vi "demo - long bad VI.vi"() -> ()   [LabVIEW 2024]
uses:
  <vilib>/Instr/_visa.llb/VISA Configure Serial Port (Instr).vi
  <vilib>/Utility/sysdir.llb/System Directory Type.ctl
  <vilib>/Analysis/NI_AALBase.lvlib
  <resource>/objmgr/daqmx.rc
  <vilib>/Utility/error.llb/DialogType.ctl
  <vilib>/sound2/lvsound2.llb/Sampling Mode.ctl
  <vilib>/sound2/lvsound2.llb/Sound Data Format.ctl
  <instrlib>/niScope/Configure/Trigger/niScope Configure Trigger Immediate.vi
  <instrlib>/niScope/Configure/Trigger/niScope Configure Trigger Digital.vi
  <instrlib>/niScope/Configure/Trigger/niScope Configure Trigger Edge.vi
  <instrlib>/niScope/Acquire/niScope Multi Read Cluster.vi
  <vilib>/Analysis/1siggen.llb/Ramp Pattern by Samples.vi
  <vilib>/DAQmx/create/channels.llb/DAQmx Create Channel (AI-Voltage-Basic).vi
  <vilib>/sound2/lvsound2.llb/Sound Output Set Volume (Single).vi
  <vilib>/DAQmx/read.llb/DAQmx Read (Analog 1D Wfm NChan NSamp).vi
  <vilib>/sound2/lvsound2.llb/Sound Output Write (DBL Single).vi
  <vilib>/DAQmx/configure/timing.llb/DAQmx Timing (Sample Clock).vi
  <vilib>/Utility/traverseref.llb/VI Scripting - Traverse.lvlib
  <vilib>/Utility/traverseref.llb/TRef TravTarget.ctl
  Serial - Settings.ctl
panel:
  out "Word count as text:":string
  out "Map of word to occurrence count:":map{string, u64}(c390)
  in  "Ignore these words:":string[](array[string])=["the", "an", "a"]
  in  "Count the words in this text:":string="Macbeth by William Shakespeare\nTomorrow, and tomorrow, and tomorrow,\nCreeps in this petty pace from day to day\nTo the last syllable of recorded time,\nAnd all our yesterdays have lighted fools\nThe way to dusty death. Out, out, brief candle!\nLife's but a walking shadow, a poor player\nThat struts and frets his hour upon the stage\nAnd then is heard no more: it is a tale\nTold by an idiot, full of sound and fury,\nSignifying nothing."
  in  "Tab Control 2":T1(tab)
  out "Numeric Result":bool
  in  "Numeric 2":i32=1
  in  "Numeric 1":i32=1
  out "String Result":bool
  in  "String 2":string="labview"
  in  "String 1":string="LabVIEW"
  out "Path Result":bool
  in  "Path 2":path=path "C:/TEST.TXT"
  in  "Path 1":path=path "c:/test.txt"
  out "Cluster Result":T2
  in  "Cluster 2":T3={"String"="test", "Numeric"=3.0, "Boolean"=TRUE}
  in  "Cluster 1":T3={"String"="test", "Numeric"=3.0, "Boolean"=TRUE}
  out "Numeric Refnum Value 2":u32
  out "Numeric Refnum Value 1":u32
  out "Refnum Result":bool
  in  "Time Stamp":timestamp
  out "Array to Scalar Result":bool[](array[boolean])
  in  "Scalar":dbl=2.0
  in  "Array":dbl[](array[numeric])=[1.0, 2.0, 3.0]
  out "Array to Array Result":bool[](array[boolean])
  in  "Array to Array 2":dbl[](array[numeric])=[1.0, 2.0, 3.0]
  in  "Array to Array 1":dbl[](array[numeric])=[1.0, 2.0, 3.0]
  in  "Tab Control":T4(tab)
  out "Max of X and Y":i32
  out "Min of X and Y":i32
  in  "Numeric Y":i32=56
  in  "Numeric X":i32=45
  out "Min String":string
  out "Max String":string
  in  "String Y":string="test ABC"
  in  "String X":string="test D"
  out "Min Path":path
  out "Max Path":path
  in  "Path Y":path=path "C:/Test1234"
  in  "Path X":path=path "C:/Test2"
  out "Maximum Cluster":T5
  out "Minimum Cluster":T5
  in  "Input Cluster Y":T5={"Numeric"=0.0, "String"="VI", "Numeric 2"=7.0}
  in  "Input Cluster X":T5={"Numeric"=1.0, "String"="test", "Numeric 2"=-3.0}
  out "Earliest Time":timestamp
  out "Latest Time":timestamp
  in  "Time Stamp Y":timestamp=timestamp(2327499010.485 s since 1904-01-01)
  in  "Time Stamp X":timestamp=timestamp(3084908797.174 s since 1904-01-01)
  out "Min Array":dbl[](array[numeric])
  out "Max Array":dbl[](array[numeric])
  in  "Array Y":dbl[](array[numeric])=[1.0, 2.0, 3.0, 4.0]
  in  "Array X":dbl[](array[numeric])=[5.0, 4.0, 3.0, 2.0, 1.0]
  in  "Device ID":u32
  in  "Stop 5":bool
  in  "Frequency":dbl=500.0
  out "Generated Sound":waveform(dbl)(graph)
  in  "Volume":dbl(slide)=50.0 scale=0.0..100.0
  in  "Server Closed":string="The server VI closed the connection."
  in  "Stop 4":bool
  out "Waveform Graph 5":dbl[](graph)
  in  "Number of Samples":i32=10000
  in  "Sample Rate":dbl=10000.0
  in  "Sample Clock Source":tag="OnboardClock"
  in  "Max Voltage":dbl=5.0
  in  "Min Voltage":dbl=-5.0
  in  "Physical Channel":tag="6363_sim/ai0"
  out "Actual Sample Rate 2":dbl=1000.0 format="%0.2f"
  out "Waveform Graph 4":waveform(dbl)[](graph)
  in  "Stop 3":bool
  out "Waveform Graph 3":dbl[](graph)
  out "current iteration 2":i32
  out "Waveform Graph 2":dbl[](graph)
  out "current iteration":i32
  out "Option String":string
  in  "Vertical Noise \n(% Range)":dbl=4.0 format="%.2f"
  in  "Board Type":u16(ring)=1 items=["PCI", "PXI", "PXIe", "USB", "AT", "PCMCIA"]
  in  "Model":u16(ring)=3 items=["NI-5102", "NI-5105", "NI-5112", "NI-5114", "NI-5122", "NI-5124", "NI-5132", "NI-5133", "NI-5142", "NI-5152", "NI-5153", "NI-5154", "NI-5160 (2CH)", "NI-5160 (4CH)", "NI-5162 (2CH)", "NI-5162 (4CH)", "NI-5170R (4CH)", "NI-5170R (8CH)", "NI-5171R (8CH)", "NI-5185", "NI-5186", "NI-5620", "NI-5621", "NI-5622", "NI-5911", "NI-5922"]
  in  "Simulate":bool
  in  "Channel(s)":string="0,1"
  in  "Vertical Range (V)":dbl=5.0 format="%.2f"
  in  "Min. Sample Rate":dbl=1000000.0 step=1000000.0 format="%#.3p"
  in  "Min. Record Length":i32=1000
  out "Waveform Graph":T6(graph)
  out "Actual Record Length":i32=1000
  out "Actual Sample Rate":dbl format="%#.3p"
  in  "Trigger Type":u16(ring)=2 items=["Edge", "Digital", "Immediate"]
  in  "Input Impedance":u32(ring) items=["1 mega ohm", "75 ohms", "50 ohms"]
  in  "Max. Input Frequency (Hz)":dbl caption="Max. Input\nFrequency (Hz)" format="%.2f"
  in  "Ref Position":dbl=50.0 format="%.1f"
  in  "Trigger Slope":i32(ring) items=["Positive", "Negative"]
  in  "Trigger Level (V)":dbl format="%.2f"
  in  "Number Of Records":i32=1 step=1
  in  "Stop 2":bool caption="stop"
  in  "Trigger Source":string(combo)="0"
  in  "Vertical Coupling":i32(ring) items=["AC", "DC", "Ground"]
  in  "Resource Name":refnum<k15>="Dev1" caption="Resource Name(s)"
  in  "Current Temperature":dbl
  in  "Threshold":dbl
  out "Alarm":bool
  out "Waveform Chart":dbl(graph)
  in  "Stop":bool
  out "XY Graph 2":cluster{"Ramp Pattern":dbl[], dbl[]}(graph)
  in  "All data":dbl[][](array[numeric])=[[-10.0, -204.0, 492.55], [-9.0, -132.17359, 359.580355], [-8.0, -87.56192, 252.88208], [-7.0, -58.99533, 169.671655], [-6.0, -39.66976, 107.11768], [-5.0, -25.71875, 62.346875], [-4.0, -15.13824, 32.45008], [-3.0, -7.01377, 14.488255], [-2.0, -0.99968, 5.49848], [-1.0, 3.00009, 2.499955], [0.0, 5.0, 2.5], [1.0, 5.00011, 2.500055], [2.0, 3.00288, -0.49832], [3.0, -0.97003, -9.487445], [4.0, -6.81056, -27.44752], [5.0, -14.15625, -57.340625], [6.0, -22.07104, -102.10472], [7.0, -28.52447, -164.647645], [8.0, -29.61888, -247.84112], [9.0, -18.51421, -354.514745]]
  out "Data written to":path
  out "XY Graph":cluster{"x axis":dbl[], "plot 1":dbl[]}[](graph)
  out "output cluster":T7
  out "timestamp":timestamp
  out "firmware":string
  out "array data":string[](array[string])
  in  "Serial Settings 2":T8={"baud rate"=9600, "data bits"=8, "parity"=enum."None", "stop bits"=10, "flow control"=0} {"flow control" items=["None"=0, "XON/XOFF"=1, "RTS/CTS"=2, "DTR/DSR"=4]; "stop bits" items=["1.0"=10, "1.5"=15, "2.0"=20]; "data bits" min=5 max=8 step=1; "baud rate" items=["75"=75, "110"=110, "134"=134, "150"=150, "300"=300, "600"=600, "1200"=1200, "1800"=1800, "2400"=2400, "4800"=4800, "7200"=7200, "9600"=9600, "14400"=14400, "19200"=19200, "28800"=28800, "38400"=38400, "56000"=56000, "57600"=57600, "115200"=115200, "128000"=128000, "230400"=230400]}
  out "bytes read 2":u32
  out "Response 2":string
  in  "delay before read (ms) 2":u32=500
  in  "VISA resource name 2":refnum<visa-resource-name>="COM3"
  in  "Serial Settings":T8={"baud rate"=9600, "data bits"=8, "parity"=enum."None", "stop bits"=10, "flow control"=0} {"flow control" items=["None"=0, "XON/XOFF"=1, "RTS/CTS"=2, "DTR/DSR"=4]; "stop bits" items=["1.0"=10, "1.5"=15, "2.0"=20]; "data bits" min=5 max=8 step=1; "baud rate" items=["75"=75, "110"=110, "134"=134, "150"=150, "300"=300, "600"=600, "1200"=1200, "1800"=1800, "2400"=2400, "4800"=4800, "7200"=7200, "9600"=9600, "14400"=14400, "19200"=19200, "28800"=28800, "38400"=38400, "56000"=56000, "57600"=57600, "115200"=115200, "128000"=128000, "230400"=230400]}
  out "bytes read":u32
  out "Response":string
  in  "delay before read (ms)":u32=500
  in  "VISA resource name":refnum<visa-resource-name>="COM3"
  # "Equal? will return TRUE if both numerics are the same value."
  # "Equal? will return TRUE if both strings are the same value. The comparison is case-sensitive, so 'LabVIEW' and 'labview' would not be considered equal."
  # "Equal? will return TRUE if both paths are the same value. The comparison is case-insensitive on some platforms (like Windows), and case-sensitive on other platforms (like Linux)."
  # "Equal? will return a cluster of Booleans with the same number of elements as the input clusters. Each Boolean will be TRUE if the corresponding elements in the clusters are the same value."
  # "Equal? will return TRUE if both refnums refer to the same control. This is the case, even if the refnums have different numeric values."
  # "Note: Control references from different sources are used for the refnum comparison. The actual value of this Time Stamp is not used in this example."
  # "When comparing arrays with arrays, Equal? will return an array of Booleans with the same number of elements as the smaller of the two input arrays. When comparing an array to a scalar, Equal? will return an array of Booleans with the same number of elements as the array."
  # "Max & Min finds the maximum and minimum of two numeric values."
  # "Max & Min compares the two strings character by character until it finds a character that has a higher ASCII numeric value. String length is not taken into account."
  # "Max & Min compares the two paths character by character until it finds a character that has a higher ASCII numeric value. Path length is not taken into account."
  # "Max & Min compares the clusters element by element, and returns clusters of the comparison results. The resulting clusters will have the same data type as the input clusters."
  # "Max & Min finds the latest time (maximum) and earliest time (minimum) of two time stamp values."
  # "Max & Min compares the arrays element by element, and returns arrays of the comparison results. The resulting arrays will be the same size as the smaller of the two input arrays."
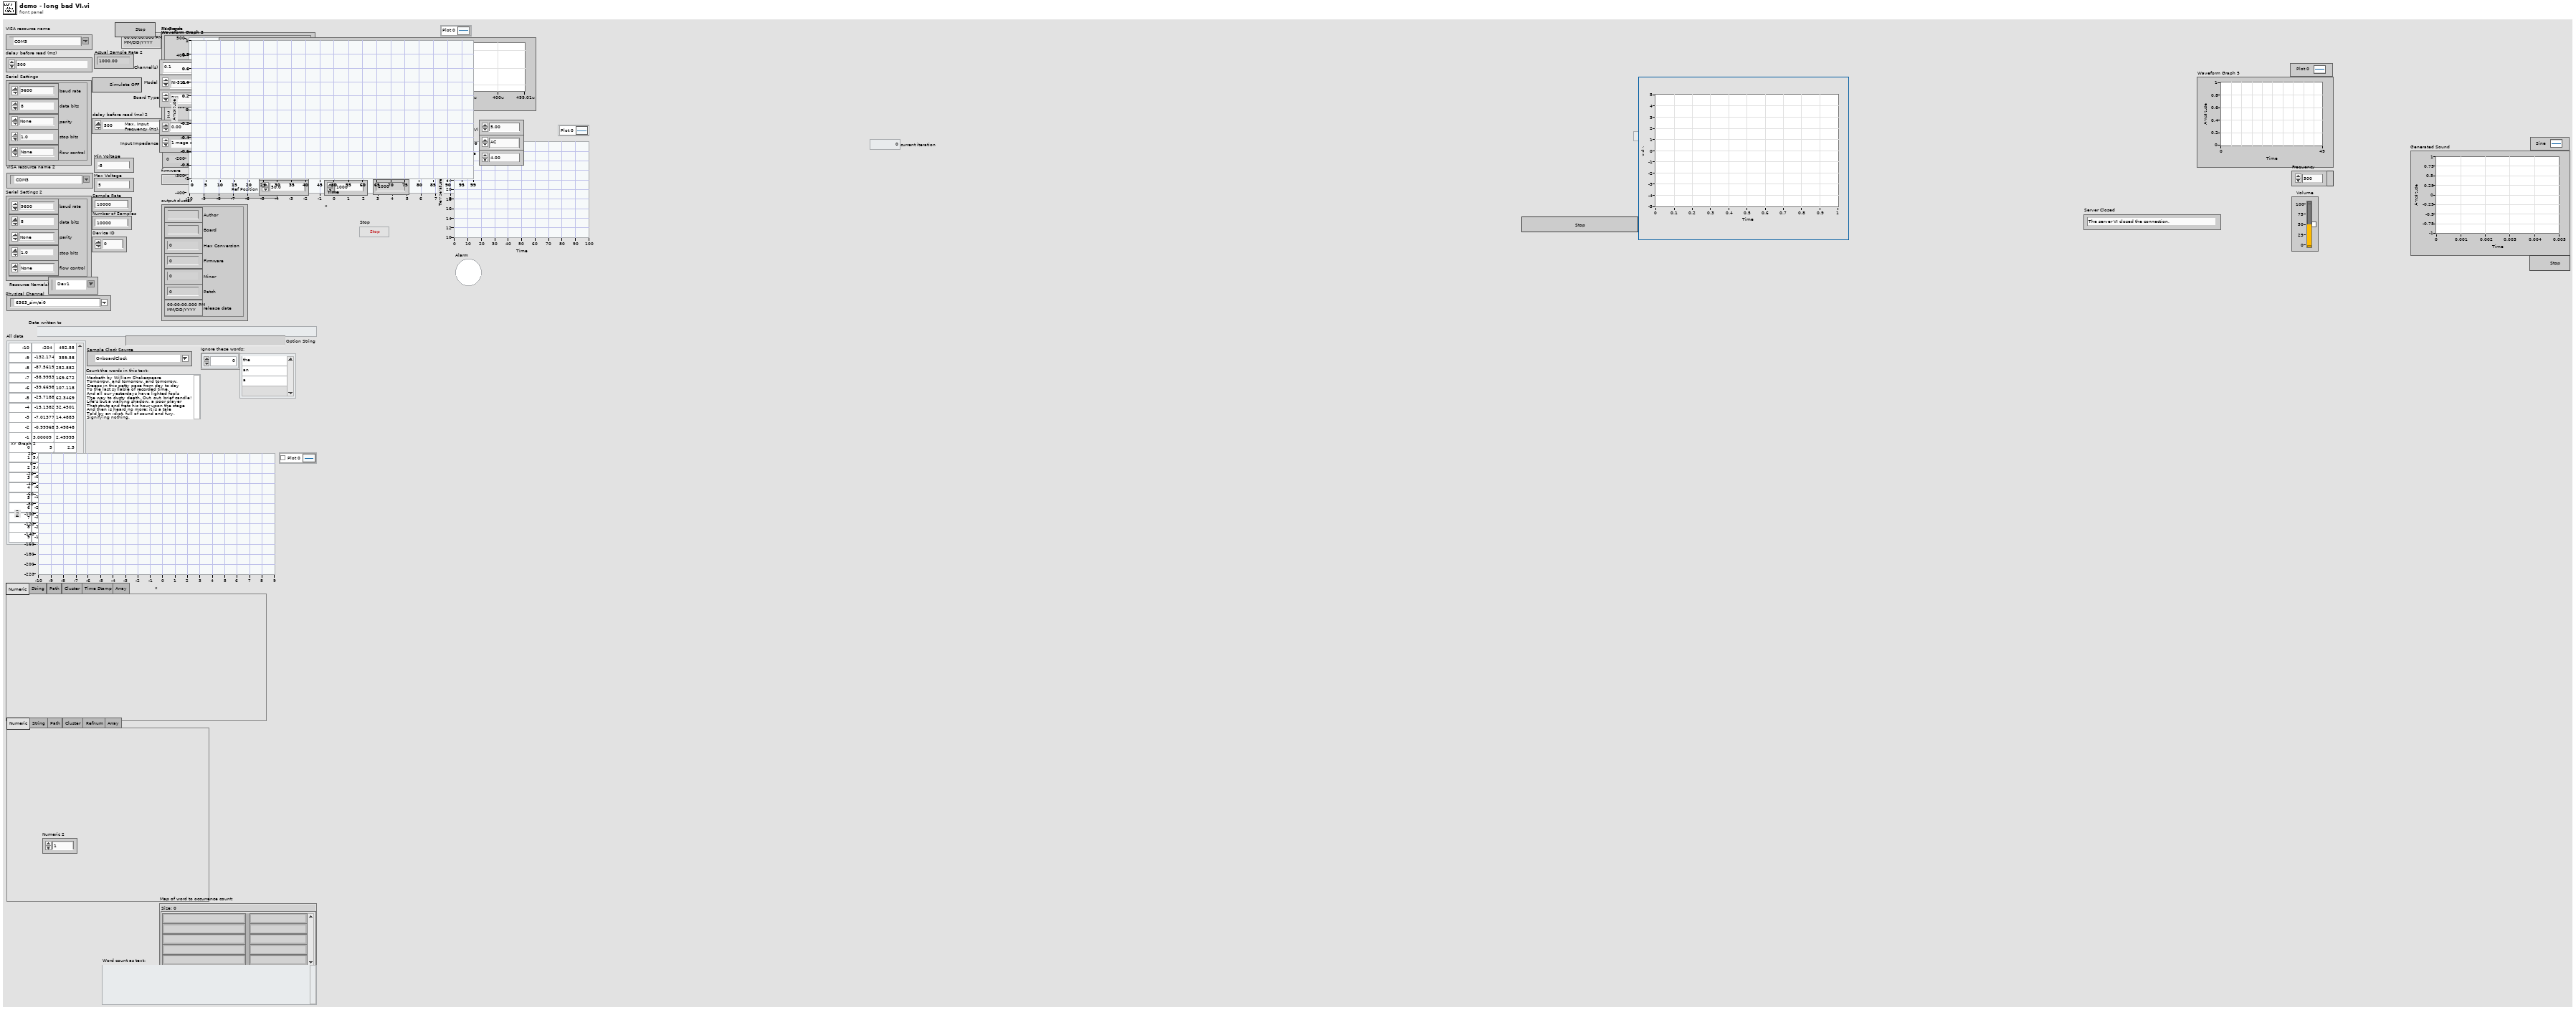
[diagram p1: front panel]
types:
  T1 = enum32{"Numeric", "String", "Path", "Cluster", "Refnum", "Array"}
  T2 = cluster{"String":bool, "Numeric":bool, "Boolean":bool}
  T3 = cluster{"String":string, "Numeric":dbl, "Boolean":bool}
  T4 = enum32{"Numeric", "String", "Path", "Cluster", "Time Stamp", "Array"}
  T5 = cluster{"Numeric":dbl, "String":string, "Numeric 2":dbl}
  T6 = cluster{"relativeInitialX":dbl, "xIncrement":dbl, "wfm":dbl[]}[]
  T7 = cluster{"Author":string, "Board":string, "Hex Conversion":u32, "Firmware":i32, "Minor":i32, "Patch":i32, "release date":timestamp}
  T8 = typedef "Serial - Settings.ctl" = cluster{"baud rate":u32, "data bits":u16, "parity":enum16{"None", "Odd", "Even", "Mark", "Space"}, "stop bits":u16, "flow control":u16}
  T9 = typedef "Sound Data Format.ctl" = cluster{"sample rate (S/s)":dbl, "number of channels":i32, "bits per sample":i32}
  T10 = typedef "TRef TravTarget.ctl" = enum16{"FP", "BD", "Other"}
  T11 = enum32{"Modify Entry only if found", "Add or Modify Entry", "Delete Entry"}
  T12 = enum16{"open", "replace", "create", "open or create", "replace or create", "replace or create with confirmation"}
  T13 = typedef "System Directory Type.ctl" = i32
  T14 = cluster{string, string, u32, i32, i32, i32, timestamp}
  T15 = typedef "DialogType.ctl" = u16
  T16 = typedef "Sampling Mode.ctl" = i32
  T17 = typedef "Sound Output Task ID.ctl" = u32
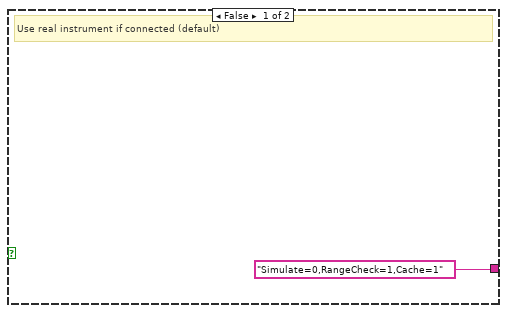
[diagram p2: hidden frame]
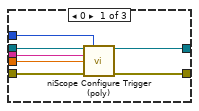
[diagram p3: hidden frame]
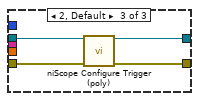
[diagram p4: hidden frame]
diagram:
  n1 = flat-sequence {
    frame #0 {
      w11 = "*IDN?\n"  # Command
      # "Report any Errors"
      # "Release Instrument"
      # "Read reply data on serial port"
      # "Wait for travel down cable"
      # "Send Command"
      # "Reserve and Configure Hardware"
      # "#vi_description \nSends a simple serial request and receives a response as as string of byte characters.\nModified NI Example.\nThetic Engineering Ltd."
      # "Use the VISA Configure Serial Port VI to configure the serial port. Send the \"*IDN?\" command with the VISA Write function. Read the response from the instrument with the VISA Read function. Note that the \"Bytes at Port\" property is used to determine how much data to read. For a single read use case, this is acceptable. For a continuous serial read, a more general approach is recommended. For an example of how to perform continuous serial communication in a loop, open the Continuous Serial Write and Read.vi in the same folder as this example."
      n2 = Unbundle By Name("Serial Settings") -> ("baud rate"=w5:u32, "data bits"=w4:u16, "parity"=w3:enum16{"None", "Odd", "Even", "Mark", "Space"}, "stop bits"=w2:u16, "flow control"=w1:u16)
      n3 = call-poly "VISA Configure Serial Port"("VISA resource name"="VISA resource name", "baud rate (9600)"=w5, "data bits (8)"=w4, "parity (0:none)"=w3, "stop bits (10: 1 bit)"=w2, "flow control (0:none)"=w1) -> ("VISA resource name out"=w20:refnum<visa-resource-name>, "error out"=w21:errorcluster)  [unwired: 3 in, 5 out]
      n4 = VISA Write(VISA resource name=w20, write buffer=w11, error in (no error)=w21) -> (VISA resource name out=w14:refnum<visa-resource-name>, error out=w16:errorcluster)  [unwired: 1 out]
      n5 = flat-sequence {
        tunnel: w16 -> [w24]
        tunnel: [w24] -> w15
        tunnel: w14 -> [w23]
        tunnel: [w23] -> w13
        tunnel: "delay before read (ms)" -> [w25]
        frame #0 {
          n6 = Wait (ms)(milliseconds to wait=w25) -> ()  [unwired: 1 out]
        }
      }
      n7 = property on="Property Node" class="Instr"(reference=w13, error in=w15) -> (reference out=w10:refnum<visa-resource-name>, error out=w9:errorcluster, "Serial Settings:Number of Bytes at Serial Port"=w7:u32)
      "bytes read" <- w7
      n8 = VISA Read(VISA resource name=w10, byte count=w7, error in (no error)=w9) -> (VISA resource name out=w18:refnum<visa-resource-name>, read buffer=→"Response":string, error out=w19:errorcluster)  [unwired: 1 out]
      n9 = VISA Close(VISA resource name=w18, error in (no error)=w19) -> (error out=w17:errorcluster)
      n10 = call <vilib>:"Simple Error Handler.vi"("error in (no error)"=w17) -> ()  [unwired: 1 in, 8 out]
    }
    frame #1 {
      w30 = 2  # column
      w31 = 1  # column
      w32 = 0  # column
      w34 = "x,function1,function2\n"  # header
      w36 = "data.csv"  # filename
      w37 = enum16{"read/write", "read-only", "write-only"}."write-only"  # access (0:read/write)
      w38 = T12."replace or create"  # operation (0:open)
      w40 = T13 1 items=["User Home"=0, "User Desktop"=1, "User Documents"=2, "User Application Data"=3, "User Preferences"=4, "User Temporary"=5, "Public Documents"=6, "Public Application Data"=7, "Public Preferences"=8, "Public Cache"=13, "System Core Libraries"=9, "System Installed Libraries"=10, "Application Files"=11, "Boot Volume Root"=12]  # system directory type
      w48 = ","  # delimiter
      w49 = "%.6f"  # format string
      # "Close the file"
      # "Write measurement data to the file, which is already a comma-separated table"
      # "Write the names of columns, at the first line, and then move the cursor to the next line"
      # "Create a file on the desktop with the right permissions and open it"
      # "Provide a 2D array (table) and convert all values to strings, separated by commas"
      # "Source data to plot of f(x) and x"
      # "#vi_description \nPlots a polynomial equation to an XY graph and stores the values into a text file.\nThetic Engineering Ltd."
      # "Create xy pairs and plot to XY graph"
      n11 = Index Array(array="All data", index (col) #1=w32, index (col) #2=w31, index (col) #3=w30) -> (element #1=w29:dbl[], element #2=w28:dbl[], element #3=w27:dbl[])  [unwired: 3 in]
      n12 = call <vilib>:"Get System Directory.vi"("system directory type"=w40) -> ("system directory"=w39:path)  [unwired: 10 in]
      n13 = Build Path(base path=w39, name or relative path=w36) -> (appended path=w33:path)
      "Data written to" <- w33
      n14 = Array To Spreadsheet String(delimiter (Tab)=w48, array="All data", 3:w49) -> (spreadsheet string=w47:string)
      n15 = Open/Create/Replace File(file path (use dialog)=w33, operation (0:open)=w38, access (0:read/write)=w37) -> (refnum out=w43:refnum<file>, error out=w44:errorcluster)  [unwired: 3 in, 1 out]
      n16 = Write to Text File(file (use dialog)=w43, text=w34, error in=w44) -> (refnum out=w45:refnum<file>, error out=w46:errorcluster)  [unwired: 1 in, 1 out]
      n17 = Write to Text File(file (use dialog)=w45, text=w47, error in=w46) -> (refnum out=w41:refnum<file>, error out=w42:errorcluster)  [unwired: 1 in, 1 out]
      n18 = Bundle("All data"=w29, "All data"=w28) -> (w52:cluster{"All data":dbl[], "All data":dbl[]})  [unwired: 1 in]
      n19 = Bundle("All data"=w29, "All data"=w27) -> (w51:cluster{"All data":dbl[], "All data":dbl[]})  [unwired: 1 in]
      n20 = Build Array(w52, w51) -> (→"XY Graph":cluster{"All data":dbl[], "All data":dbl[]}[])
      n21 = Close File(refnum=w41, error in=w42) -> (error out=w35:errorcluster)  [unwired: 1 out]
      n22 = call <vilib>:"Simple Error Handler.vi"("error in (no error)"=w35) -> ()  [unwired: 4 in, 5 out]
    }
    frame #2 {
      w53 = TRUE  # exclude end?
      w57 = 20  # samples
      w58 = 10.0  # end
      w59 = -10.0  # start
      # "#vi_description \nPlots a polynomial equation to an XY graph, demonstrating the use of a formula node.\nThetic Engineering Ltd."
      # "Create xy pairs and plot to XY graph"
      # "Generate integer values from -10 to 10"
      # "target equation (screenshot)"
      n23 = call-poly <vilib>:"Ramp Pattern.vi"("exclude end?"=w53, "start"=w59, "end"=w58, "samples"=w57) -> ("Ramp Pattern"=w55:dbl[])  [unwired: 6 in, 1 out]
      n24 = for {
        tunnel: w55 -> [w61] mode=indexing
        tunnel: [w60] -> w56 mode=indexing
        # "Auto-indexing For Loop will produce a result for each value of x"
        n25 = formula code="fx = 10**-5*x**7 + 10**-4*x**4 - x**2 + x + 5;"("x"=w61) -> ("fx"=w60:dbl)
      }
      n26 = Bundle("Ramp Pattern"=w55, w56) -> (→"XY Graph 2":cluster{"Ramp Pattern":dbl[], dbl[]})  [unwired: 1 in]
    }
    frame #3 {
      # "#vi_description \nChecks if temperature exceeds the threshold, in Celsius\nThetic Engineering Ltd."
      n27 = while {
        stop <- "Stop" stop-if-true
        w62 = u32 100  # millisecond multiple
        # "Checks if Temperature exceeds threshold, in Celsius"
        n28 = Wait Until Next ms Multiple(millisecond multiple=w62) -> ()  [unwired: 1 out]
        n29 = Greater Or Equal?(x="Current Temperature", y="Threshold") -> (x >= y?=→"Alarm":bool)
        "Waveform Chart" <- "Current Temperature"
      }
    }
    frame #4 {
      w74 = FALSE  # Reset Device
      # "#vi_description \nSimulates a 2 ch digitizer and plots the graph.  This is an NI example from NI-SCOPE that has been modifed.\nThetic Engineering Ltd."
      # "11"
      # "1. Form a string that will be used to initialize the oscilloscope. The simulation string should look like \"Simulate=1,DriverSetup=Model:5122;BoardType:PXI\".\n2. Open a session to the oscilloscope. Use init with options and pass the string formed in step 1.\n3. Configure the vertical parameters such as input range, offset and coupling.\n       For more information regarding channel names, refer to Channel String Syntax in the NI High-Speed Digitizers Help.\n4. Configure the channel characteristics such as input impedance and bandwidth.\n5. Configure the horizontal parameters such as sampling rate and number of samples to acquire.\n6. Configure the trigger. All oscilloscopes support immediate triggering. Choose between immediate, analog or digital.\n7. Use the Read function to Initiate the acquisition, wait until it finishes and fetch the acquired data. In simulation mode a Sine will be returned for channel 0 and a Square for channel 1.\n8. Query for the actual (coerced) record length.\n9. Query for the actual (coerced) sampling rate.\n10. Check for errors, and stop if any occurred. Also stop if the \"Stop\" button is clicked.\n11. Close the session and display any errors that might have occurred."
      # "2"
      n30 = case shown="True" "Simulate" {
        tunnel: ["Simulate=0,RangeCheck=1,Cache=1" ("option string") w91] -> w67
        frame False {
          # "Use real instrument if connected (default)"
        }
        frame True {
          (unwired) "BoardType:PCI"  # Board Type Format
          (unwired) "Model:5102;"  # Model String Format
          w94 = "Simulate=1,DriverSetup=Noise:"  # General Setup
          # "1"
          # "Generate option string to enable NI-SCOPE simulation"
          n31 = property on="Model" class="Ring (strict)"() -> ("Strings []"=w90:string[])  [unwired: 2 in, 2 out]
          n32 = property on="Board Type" class="Ring (strict)"() -> ("Strings []"=w82:string[])  [unwired: 2 in, 2 out]
          n33 = Index Array(array=w90, index="Model") -> (element=w88:string)
          n34 = Index Array(array=w82, index="Board Type") -> (element=w80:string)
          n35 = String Subset(string=w88, offset (0)=3 ("Offset (0)")) -> (substring=w85:string)  [unwired: 1 out]
          n36 = Concatenate Strings("BoardType:" ("Board Type Format"), w80) -> (w78:string)
          n37 = Concatenate Strings("Model:" ("String"), w85, ";" ("String")) -> (w86:string)
          n38 = Number To Fractional String(use system decimal point (T)=FALSE ("Use System Decimal Point (T)"), number="Vertical Noise \n(% Range)") -> (F-format string=w93:string)  [unwired: 2 out]
          n39 = Concatenate Strings(w94, w93, ";", w86, w78) -> (w91:string)
        }
      }
      "Option String" <- w67
      n40 = call <instrlib>:"niScope Initialize With Options.vi"("resource name"="Resource Name", "option string"=w67, "reset device"=w74) -> ("instrument handle"=w72:refnum<k15>, "error out"=w71:errorcluster)  [unwired: 2 in, 9 out]
      n41 = while {
        tunnel: w72 -> [w98]
        tunnel: [w104] -> w70
        shift-right: [w103] -> w69
        shift-left: w71 -> [w97]
        stop <- w105 stop-if-true
        # "10"
        # "9"
        # "8"
        # "6"
        # "7"
        # "5"
        # "4"
        # "3"
        n42 = call <instrlib>:"niScope Configure Vertical.vi"("instrument handle"=w98, "vertical coupling"="Vertical Coupling", "channels"="Channel(s)", "vertical range"="Vertical Range (V)", "error in"=w97) -> ("instrument handle out"=w123:refnum<k15>, "error out"=w122:errorcluster)  [unwired: 3 in, 6 out]
        n43 = call <instrlib>:"niScope Configure Chan Characteristics.vi"("instrument handle"=w123, "channels"="Channel(s)", "input impedance"="Input Impedance", "maximum input frequency"="Max. Input Frequency (Hz)", "error in"=w122) -> ("instrument handle out"=w120:refnum<k15>, "error out"=w121:errorcluster)  [unwired: 9 out]
        n44 = call <instrlib>:"niScope Configure Horizontal Timing.vi"("instrument handle"=w120, "number of records"="Number Of Records", "min sample rate"="Min. Sample Rate", "reference position"="Ref Position", "error in"=w121, "min record length"="Min. Record Length") -> ("instrument handle out"=w116:refnum<k15>, "error out"=w117:errorcluster)  [unwired: 1 in, 7 out]
        n45 = case "Trigger Selection" shown="1" "Trigger Type" {
          tunnel: w117 -> [w137 w143 w147]
          tunnel: [w133 w139 w144] -> w109
          tunnel: w116 -> [w136 w142 w146]
          tunnel: [w134 w140 w145] -> w110
          tunnel: "Trigger Source" -> [w135 w141 _]
          tunnel: "Trigger Level (V)" -> [w132 _ _]
          tunnel: "Trigger Slope" -> [w131 w138 _]
          frame 0 {
            n46 = call-poly <instrlib>:"niScope Configure Trigger (poly).vi"("instrument handle"=w136, "trigger slope"=w131, "trigger source"=w135, "trigger level"=w132, "error in"=w137) -> ("instrument handle out"=w134:refnum<k15>, "error out"=w133:errorcluster)  [unwired: 3 in, 6 out]
          }
          frame 1 {
            n47 = call-poly <instrlib>:"niScope Configure Trigger (poly).vi"("instrument handle"=w142, "trigger slope"=w138, "trigger source"=w141, "error in"=w143) -> ("instrument handle out"=w140:refnum<k15>, "error out"=w139:errorcluster)  [unwired: 2 in, 8 out]
          }
          frame 2, Default {
            n48 = call-poly <instrlib>:"niScope Configure Trigger (poly).vi"("instrument handle"=w146, "error in"=w147) -> ("instrument handle out"=w145:refnum<k15>, "error out"=w144:errorcluster)  [unwired: 12 out]
          }
        }
        n49 = call-poly <instrlib>:"niScope Read (poly).vi"("error in"=w109, "channels"="Channel(s)", "instrument handle"=w110) -> ("error out"=w107:errorcluster, "waveform"=→"Waveform Graph":T6, "instrument handle out"=w108:refnum<k15>)  [unwired: 2 in, 4 out]
        n50 = call <instrlib>:"niScope Actual Record Length.vi"("instrument handle"=w108, "error in"=w107) -> ("instrument handle out"=w127:refnum<k15>, "actual record length"=→"Actual Record Length":i32, "error out"=w126:errorcluster)  [unwired: 11 out]
        n51 = Wait (ms)(milliseconds to wait=u32 20 ("Milliseconds To Wait")) -> ()  [unwired: 1 out]
        n52 = call <instrlib>:"niScope Sample Rate.vi"("instrument handle"=w127, "error in"=w126) -> ("instrument handle out"=w104:refnum<k15>, "actual sample rate"=→"Actual Sample Rate":dbl, "error out"=w103:errorcluster)  [unwired: 11 out]
        n53 = Or(x=w103, y="Stop 2") -> (x .or. y?=w105:bool)
      }
      n54 = call <instrlib>:"niScope Close.vi"("instrument handle"=w70, "error in"=w69) -> ("error out"=w73:errorcluster)  [unwired: 13 out]
      n55 = call <vilib>:"Simple Error Handler.vi"("error in (no error)"=w73) -> ()  [unwired: 1 in, 8 out]
    }
    frame #5 {
      # "#vi_description \nPlot a finite sine wave onto a waveform graph\nThetic Engineering Ltd."
      n56 = for {
        N: 100 -> [_]
        tunnel: [w150] -> w148 mode=indexing
        i -> [w151]
        w152 = u32 10  # ms multiple
        w153 = 3  # y
        # "For Loop"
        n57 = Divide(x=w151, y=w153) -> (x/y=w154:dbl)
        n58 = Sine(x=w154) -> (sin(x)=w150:dbl)
        n59 = Wait Until Next ms Multiple(millisecond multiple=w152) -> ()  [unwired: 1 out]
        "current iteration" <- w151
      }
      "Waveform Graph 2" <- w148
    }
    frame #6 {
    }
    frame #7 {
      w164 = "%3s,%11s,%x,%1d.%1d.%1d.%<%Y%m%dT%H%M%S>T"  # format string
      w167 = "%<%Y%m%dT%H%M%S>T"  # format string
      w170 = "[0-9].[0-9].[0-9]."  # regular expression
      w172 = 3  # index
      w168 = ","  # delimiter
      w183 = "*IDN?\n"  # Command
      # "Single stage method"
      # "Multi-stage method"
      # "Report any Errors"
      # "Release Instrument"
      # "Read reply data on serial port"
      # "Wait for travel down cable"
      # "Send Command"
      # "Reserve and Configure Hardware"
      # "#vi_description \nSends a simple serial request and receives a response as as string of byte characters.\nModified NI Example.\nThetic Engineering Ltd."
      n60 = Unbundle By Name("Serial Settings 2") -> ("baud rate"=w178:u32, "data bits"=w177:u16, "parity"=w176:enum16{"None", "Odd", "Even", "Mark", "Space"}, "stop bits"=w175:u16, "flow control"=w174:u16)
      n61 = call-poly "VISA Configure Serial Port"("VISA resource name"="VISA resource name 2", "baud rate (9600)"=w178, "data bits (8)"=w177, "parity (0:none)"=w176, "stop bits (10: 1 bit)"=w175, "flow control (0:none)"=w174) -> ("VISA resource name out"=w192:refnum<visa-resource-name>, "error out"=w193:errorcluster)  [unwired: 3 in, 5 out]
      n62 = VISA Write(VISA resource name=w192, write buffer=w183, error in (no error)=w193) -> (VISA resource name out=w186:refnum<visa-resource-name>, error out=w188:errorcluster)  [unwired: 1 out]
      n63 = flat-sequence {
        tunnel: w188 -> [w196]
        tunnel: [w196] -> w187
        tunnel: w186 -> [w195]
        tunnel: [w195] -> w185
        tunnel: "delay before read (ms) 2" -> [w197]
        frame #0 {
          n64 = Wait (ms)(milliseconds to wait=w197) -> ()  [unwired: 1 out]
        }
      }
      n65 = property on="Property Node" class="Instr"(reference=w185, error in=w187) -> (reference out=w182:refnum<visa-resource-name>, error out=w181:errorcluster, "Serial Settings:Number of Bytes at Serial Port"=w180:u32)
      "bytes read 2" <- w180
      n66 = VISA Read(VISA resource name=w182, byte count=w180, error in (no error)=w181) -> (VISA resource name out=w190:refnum<visa-resource-name>, read buffer=w156:string, error out=w191:errorcluster)  [unwired: 1 out]
      "Response 2" <- w156
      n67 = call <vilib>:"Delimited String to 1D String Array.vi"("delimiter"=w168, "delimited string"=w156) -> ("string array"=w173:string[])  [unwired: 9 in]
      "array data" <- w173
      n68 = VISA Close(VISA resource name=w190, error in (no error)=w191) -> (error out=w189:errorcluster)
      n69 = Index Array "Index Array"(array=w173, index=w172) -> (element=w171:string)
      n70 = Match Pattern(string=w171, regular expression=w170) -> (match substring=→"firmware":string, after substring=w166:string)  [unwired: 1 in, 2 out]
      n71 = call <vilib>:"Simple Error Handler.vi"("error in (no error)"=w189) -> ()  [unwired: 1 in, 8 out]
      n72 = Scan From String "Scan From String"(format string=w167, input string=w166) -> (output 1=→"timestamp":timestamp)  [unwired: 3 in, 3 out]
      n73 = Scan From String "Scan From String"(format string=w164, input string=w156) -> (output 1=w163:string, output 2=w162:string, output 3=w161:u32, output 4=w160:i32, output 5=w159:i32, output 6=w158:i32, output 7=w157:timestamp)  [unwired: 9 in, 3 out]
      n74 = Bundle(w163, w162, w161, w160, w159, w158, w157) -> (→"output cluster":T14)  [unwired: 1 in]
    }
    frame #8 {
      # "#vi_description \nPlot a finite sine wave onto a waveform graph\nThetic Engineering Ltd."
      n75 = for {
        N: 100 -> [_]
        tunnel: [w200] -> w198 mode=indexing
        i -> [w201]
        w202 = u32 10  # ms multiple
        w203 = 3  # y
        # "For Loop"
        n76 = Divide(x=w201, y=w203) -> (x/y=w204:dbl)
        n77 = Sine(x=w204) -> (sin(x)=w200:dbl)
        n78 = Wait Until Next ms Multiple(millisecond multiple=w202) -> ()  [unwired: 1 out]
        "current iteration 2" <- w201
      }
      "Waveform Graph 3" <- w198
    }
    frame #9 {
      w215 = -1 items=["default"=-1, "RSE"=10083, "NRSE"=10078, "Differential"=10106, "Pseudodifferential"=12529]  # Terminal Configuration
      w205 = T15 3 items=["no dialog", "OK message", "continue or stop message", "OK message + warnings", "continue/stop + warnings"] ("type of dialog (OK msg:1)")
      w225 = 10123 items=["Finite Samples"=10178, "Continuous Samples"=10123, "Hardware Timed Single Point"=12522]  # Sample Mode
      # "#vi_description \nPlot buffered DAQmx data onto a waveform graph until the user presses stop or an error has occurred.\nThetic Engineering Ltd."
      # "Acquire Data"
      # "Timing Settings"
      # "Channel Settings"
      n79 = call-poly <vilib>:"DAQmx Create Virtual Channel.vi"("maximum value"="Max Voltage", "minimum value"="Min Voltage", "input terminal configuration"=w215, "physical channels"="Physical Channel") -> ("task out"=w223:refnum<k21>, "error out"=w224:errorcluster)  [unwired: 10 in]
      n80 = call-poly <vilib>:"DAQmx Timing.vi"("task/channels in"=w223, "sample mode"=w225, "samples per channel"="Number of Samples", "rate"="Sample Rate", "source"="Sample Clock Source", "error in"=w224) -> ("task out"=w227:refnum<k21>, "error out"=w226:errorcluster)  [unwired: 8 in]
      n81 = property class="DAQmx Timing"(reference=w227, error in=w226) -> (reference out=w222:refnum<k21>, error out=w221:errorcluster, "SampClk.Rate"=→"Actual Sample Rate 2":dbl)
      n82 = call <vilib>:"DAQmx Start Task.vi"("task/channels in"=w222, "error in"=w221) -> ("task out"=w220:refnum<k21>, "error out"=w219:errorcluster)  [unwired: 12 in]
      n83 = while {
        tunnel: w220 -> [w236]
        tunnel: w219 -> [w235]
        tunnel: [w234] -> w209
        tunnel: [w231] -> w208
        tunnel: "Number of Samples" -> [w228]
        stop <- w229 stop-if-true
        n84 = call-poly <vilib>:"DAQmx Read.vi"("task/channels in"=w236, "number of samples per channel"=w228, "error in"=w235) -> ("task out"=w234:refnum<k21>, "data"=→"Waveform Graph 4":waveform(dbl)[], "error out"=w231:errorcluster)  [unwired: 10 in]
        n85 = Unbundle By Name(w231) -> ("status"=w230:bool)
        n86 = Or(x=w230, y="Stop 3") -> (x .or. y?=w229:bool)
      }
      n87 = call <vilib>:"DAQmx Stop Task.vi"("task/channels in"=w209, "error in"=w208) -> ("task out"=w206:refnum<k21>, "error out"=w207:errorcluster)  [unwired: 12 in]
      n88 = call <vilib>:"DAQmx Clear Task.vi"("task in"=w206, "error in"=w207) -> ("error out"=w218:errorcluster)  [unwired: 13 in]
      n89 = call <vilib>:"Simple Error Handler.vi"("type of dialog (OK msg:1)"=w205, "error in (no error)"=w218) -> ()  [unwired: 3 in, 5 out]
    }
    frame #10 {
      w237 = u16 6340  # port
      w238 = "localhost"  # address
      # "Use TCP Write to send a single character to the server to indicate that the client has stopped. TCP Close Connection closes the connection when the user clicks Stop or an error occurs.\n\nTCP Close Connection will return certain error codes if the server has already disconnected. Because these errors are expected, ignore them and instead pop up a dialog indicating that the server closed the connection."
      # "Read the data on the specified connection. The first TCP Read function acquires the size of the data, and the second TCP Read function reads the data itself if the size of the data (specified by the server) is greater than zero."
      # "Open a TCP connection with the TCP Open Connection function. Note that the port must match the one specified in Simple TCP - Server.vi."
      n90 = TCP Open Connection(address=w238, remote port or service name=w237) -> (connection ID=w247:refnum<k5>, error out=w246:errorcluster)  [unwired: 3 in]
      n91 = while {
        tunnel: w246 -> [w257]
        tunnel: w247 -> [w258]
        tunnel: [w253] -> w244
        tunnel: [w252] -> w242
        stop <- w254 stop-if-true
        w256 = 4  # bytes to read
        # "TCP Client Loop"
        n92 = TCP Read(connection ID=w258, bytes to read=w256, error in (no error)=w257, 9:1000 ("timeout ms (25000)")) -> (connection ID out=w260:refnum<k5>, data out=w261:string, error out=w259:errorcluster)  [unwired: 1 in]
        n93 = Type Cast(type=w256, x=w261) -> (*(type *) &x=w251:i32)
        n94 = case shown="Default" w251 {
          selector: w251 -> [_ w264]
          tunnel: w260 -> [w263 w271]
          tunnel: w259 -> [w262 w270]
          tunnel: [w263 w267] -> w253
          tunnel: [w262 w266] -> w252
          frame ..0 {
            # "The server has not written any data"
          }
          frame Default {
            n95 = TCP Read(connection ID=w271, bytes to read=w264, error in (no error)=w270) -> (connection ID out=w267:refnum<k5>, data out=w265:string, error out=w266:errorcluster)  [unwired: 2 in]
            n96 = Type Cast(type=dbl[] [] ("chart"), x=w265) -> (*(type *) &x=→"Waveform Graph 5":dbl[])
          }
        }
        n97 = Or(x=w252, y="Stop 4") -> (x .or. y?=w254:bool)
      }
      n98 = TCP Write(connection ID=w244, data in="Q", error in (no error)=w242) -> (connection ID out=w245:refnum<k5>, error out=w243:errorcluster)  [unwired: 2 out]
      n99 = TCP Close Connection(connection ID=w245, error in (no error)=w243) -> (error out=w240:errorcluster)  [unwired: 1 in, 1 out]
      n100 = case shown="Error 62, 64, 66" w240 {
        selector: w240 -> [w248 _]
        tunnel: [w248 _] -> w239
        frame #0 {
        }
        frame #1 {
          n101 = One Button Dialog(message="Server Closed") -> ()  [unwired: 1 in, 1 out]
        }
      }
      n102 = call <vilib>:"Simple Error Handler.vi"("error in (no error)"=w239) -> ()  [unwired: 4 in, 5 out]
    }
    frame #11 {
      w275 = T16 1 items=["Finite Samples", "Continuous Samples"] ("sample mode")
      # "Configure the sound output for continuous generation."
      # "Clear the Sound Output task."
      n103 = call <vilib>:"Sound Output Configure.vi"("number of samples/ch"=5000 ("Number of Samples/ch"), "sample mode"=w275, "sound format"=T9 {"sample rate (S/s)"=44100.0, "number of channels"=2, "bits per sample"=16} ("Sound Format"), "device ID"="Device ID") -> ("error out"=w280:errorcluster, "task ID"=w279:T17)  [unwired: 6 in]
      n104 = while {
        tunnel: w279 -> [w288]
        tunnel: [w293] -> w277
        tunnel: w280 -> [w290]
        tunnel: [w286] -> w278
        stop <- w291 stop-if-true
        # "Set the volume of the output device to the specified value."
        # "Generate the sine waveform with specified frequency and amplitude of 1. Display the generated data in the graph. Play the generated waveform by writing the data to the output device."
        # "Generate Sound"
        n105 = call-poly <vilib>:"Sound Output Set Volume.vi"("error in (no error)"=w290, "volume"="Volume", "task ID"=w288) -> ("error out"=w284:errorcluster, "task ID out"=w289:T17)  [unwired: 7 in]
        n106 = call "Simulate Signal"("Frequency"="Frequency", "error in (no error)"=w284) -> ("Sine"=w282:dynamicdata, "error out"=w283:errorcluster)  [unwired: 12 in]
        n107 = call "Convert from Dynamic Data"("Dynamic Data Type"=w282) -> ("Waveform"=w285:waveform(dbl))  [unwired: 3 in]
        "Generated Sound" <- w285
        n108 = call-poly <vilib>:"Sound Output Write.vi"("error in (no error)"=w283, "data"=w285, "task ID"=w289) -> ("error out"=w286:errorcluster, "task ID out"=w293:T17)  [unwired: 7 in]
        n109 = Or(x=w286, y="Stop 5") -> (x .or. y?=w291:bool)
      }
      n110 = call <vilib>:"Sound Output Clear.vi"("error in (no error)"=w278, "task ID"=w277) -> ("error out"=w273:errorcluster)  [unwired: 9 in]
      n111 = call <vilib>:"Simple Error Handler.vi"("error in (no error)"=w273) -> ()  [unwired: 4 in, 5 out]
    }
    frame #12 {
      # "Max & Min finds the latest time (maximum) and earliest time (minimum) of two time stamp values."
      # "Max & Min compares the clusters element by element, and returns clusters of the comparison results. The resulting clusters will have the same data type as the input clusters."
      # "Max & Min compares the two paths character by character until it finds a character that has a higher ASCII numeric value. Path length is not taken into account."
      # "Max & Min compares the two strings character by character until it finds a character that has a higher ASCII numeric value. String length is not taken into account."
      # "Max & Min compares the arrays element by element, and returns arrays of the comparison results. The resulting arrays will be the same size as the smaller of the two input arrays."
      # "Max & Min finds the maximum and minimum of two numeric values"
      n112 = Max & Min(x="Path X", y="Path Y") -> (max(x,y)=→"Max Path":path, min(x,y)=→"Min Path":path)
      n113 = Max & Min(x="String X", y="String Y") -> (max(x,y)=→"Max String":string, min(x,y)=→"Min String":string)
      n114 = Max & Min(x="Numeric X", y="Numeric Y") -> (max(x,y)=→"Max of X and Y":i32, min(x,y)=→"Min of X and Y":i32)
      n115 = Max & Min(x="Input Cluster X", y="Input Cluster Y") -> (max(x,y)=→"Maximum Cluster":T5, min(x,y)=→"Minimum Cluster":T5)
      n116 = Max & Min(x="Time Stamp X", y="Time Stamp Y") -> (max(x,y)=→"Latest Time":timestamp, min(x,y)=→"Earliest Time":timestamp)
      n117 = Max & Min(x="Array X", y="Array Y") -> (max(x,y)=→"Max Array":dbl[], min(x,y)=→"Min Array":dbl[])
    }
    frame #13 {
      w321 = u32 0  # U32
      w323 = u32 0  # U32
      # "When comparing arrays with arrays, Equal? will return an array of Booleans with the same number of elements as the smaller of the two input arrays. When comparing an array to a scalar, Equal? will return an array of Booleans with the same number of elements as the array.\n\nNote: To compare two arrays as aggregates, right-click the Equal? function and select Comparison Mode > Compare Aggregates. This will cause the Equal? function to return a single Boolean with a value of TRUE if the arrays are the same size, and each corresponding array element is equal."
      # "Equal? will return TRUE if both refnums refer to the same control. This is the case, even if the refnums have different numeric values."
      # "Equal? will return TRUE if both paths are the same value. The comparison is case-insensitive on some platforms (like Windows), and case-sensitive on other platforms (like Linux)."
      # "Equal? will return a cluster of Booleans with the same number of elements as the input clusters. Each Boolean will be TRUE if the corresponding elements in the clusters are the same value."
      # "Equal? will return TRUE if both strings are the same value. The comparison is case-sensitive, so 'LabVIEW' and 'labview' would not be considered equal."
      # "Equal? will return TRUE if both numerics are the same value."
      n118 = Equal?(x="Path 1", y="Path 2") -> (x = y?=→"Path Result":bool)
      n119 = Equal?(x="Numeric 1", y="Numeric 2") -> (x = y?=→"Numeric Result":bool)
      n120 = Equal?(x="String 1", y="String 2") -> (x = y?=→"String Result":bool)
      n121 = Equal?(x="Cluster 1", y="Cluster 2") -> (x = y?=→"Cluster Result":T2)
      n122 = control-ref of="This VI"() -> (w328:refnum<vi>)
      n123 = call <vilib>:"Traverse for GObjects.vi"("Traverse Target"=TRef_TravTarget."FP", "Class Name"="AbsTime", "VI Refnum"=w328) -> ("error out"=w325:errorcluster, "References"=w326:refnum<vi>[])  [unwired: 5 in, 2 out]
      n124 = control-ref of="Time Stamp"() -> (w320:refnum<vi>)
      n125 = Index Array(array=w326) -> (element=w324:refnum<vi>)  [unwired: 1 in]
      n126 = call <vilib>:"Simple Error Handler.vi"("error in (no error)"=w325) -> ()  [unwired: 4 in, 5 out]
      n127 = Type Cast(type=w323, x=w324) -> (*(type *) &x=→"Numeric Refnum Value 2":u32)
      n128 = Type Cast(type=w321, x=w320) -> (*(type *) &x=→"Numeric Refnum Value 1":u32)
      n129 = Equal?(x=w320, y=w324) -> (x = y?=→"Refnum Result":bool)
      n130 = Equal?(x="Array to Array 1", y="Array to Array 2") -> (x = y?=→"Array to Array Result":bool[])
      n131 = Equal?(x="Array", y="Scalar") -> (x = y?=→"Array to Scalar Result":bool[])
    }
    frame #14 {
      w353 = map{string, u64} {}  # map constant
      w355 = 0  # offset past token
      # "Parse the words out of the string and add each one to the map."
      # "Iterate over the map to produce a formatted string."
      # "Remove the ignored words."
      n132 = while {
        tunnel: "Count the words in this text:" -> [w373]
        shift-left: w355 -> [w374]
        shift-right: [w365] -> _
        shift-right: [w368] -> w352
        shift-left: w353 -> [w367]
        i -> [w371]
        stop <- w372 stop-if-true
        # "Parse each word."
        n133 = Not Equal To 0?(x=w371) -> (x != 0?=w370:bool)
        n134 = Scan String For Tokens(4:w370, 8:w374, 9:w373) -> (1:w369:string, 2:w365:i32)  [unwired: 3 in, 2 out]
        n135 = To Lower Case(string=w369) -> (all lower case string=w366:string)
        n136 = in-place {
          n137 = in-place-map #1(w367, w366) -> (w377:u64)  [unwired: 1 in, 1 out]
          n138 = Increment(x=w377) -> (x+1=w376:u64)
          n139 = in-place-map #1(w376, T11."Add or Modify Entry" ("action")) -> (w368:map{string, u64})  [unwired: 2 out]
        }
        n140 = Less Than 0?(x=w365) -> (x < 0?=w372:bool)
      }
      n141 = for {
        tunnel: "Ignore these words:" -> [w363] mode=indexing
        shift-right: [w362] -> w350
        shift-left: w352 -> [w364]
        n142 = Remove From Map(10:w363, 11:w364) -> (3:w362:map{string, u64})  [unwired: 2 out]
      }
      "Map of word to occurrence count:" <- w350
      n143 = for {
        tunnel: w350 -> [w361] mode=indexing
        shift-right: [w359] -> w348
        shift-left: "" -> [w358]
        n144 = Unbundle By Name(w361) -> ("word"=w357:string, "count"=w356:u64)
        n145 = Format Into String(format string="%s: %d\\n", initial string=w358, w357, w356) -> (resulting string=w359:string)  [unwired: 1 in, 1 out]
      }
      "Word count as text:" <- w348
    }
  }
